vi "Calculate Curve Distance.vi"(9 "error in (no error)":errorcluster, 11 "Points":T1[](array[typedef])) -> (1 "error out":errorcluster, 2 "Length":dbl, 3 "Points Out":T1[](array[typedef]), 5 "Distance vs t":cluster{"t":dbl[], "Distance":dbl[]})   [LabVIEW 2019, in "Tool Path.lvclass"]
uses:
  Tool Path.lvclass
  Parse/PathCommands/Point.ctl
  Parse/PathCommands/PathCommands.lvclass
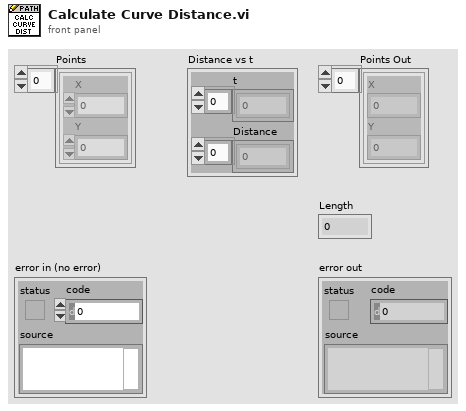
[diagram p1: front panel]
types:
  T1 = typedef "PathCommands.lvclass/Point.ctl" = cluster{"X":dbl, "Y":dbl}
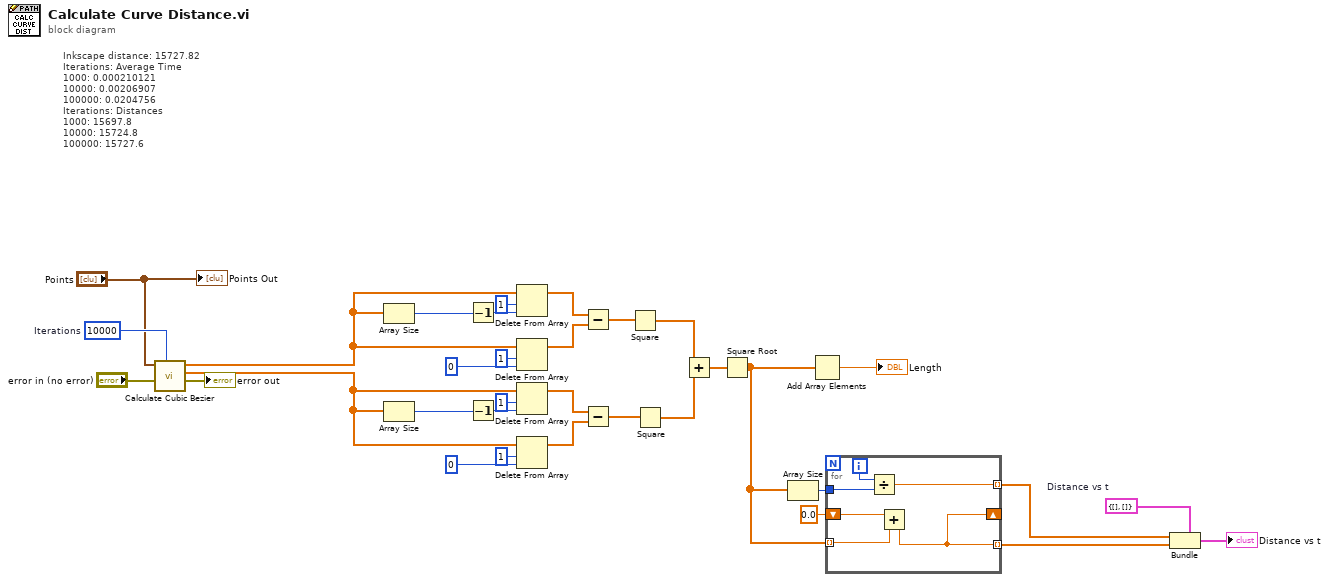
[diagram p0: block diagram]
diagram:
  w1 = cluster{"t":dbl[], "Distance":dbl[]} {"t"=[], "Distance"=[]}  # Distance vs t
  w19 = 10000  # Iterations
  # "Inkscape distance: 15727.82\nIterations: Average Time\n1000: 0.000210121\n10000: 0.00206907\n100000: 0.0204756\nIterations: Distances\n1000: 15697.8\n10000: 15724.8\n100000: 15727.6"
  n1 = call "Calculate Cubic Bezier.vi"("Iterations"=w19, "error in (no error)"="error in (no error)", "Points"="Points") -> ("error out"=→"error out":errorcluster, "Y"=w9:dbl[], "X"=w10:dbl[])  [unwired: 6 in]
  n2 = Array Size(array=w10) -> (size(s)=w33:i32)
  n3 = Array Size(array=w9) -> (size(s)=w23:i32)
  n4 = Decrement(x=w33) -> (x-1=w32:i32)
  n5 = Decrement(x=w23) -> (x-1=w24:i32)
  n6 = Delete From Array(array=w10, length=1, index=w32) -> (array with subset deleted=w18:dbl[])  [unwired: 1 out]
  n7 = Delete From Array(array=w10, length=1, index=0) -> (array with subset deleted=w17:dbl[])  [unwired: 1 out]
  n8 = Delete From Array(array=w9, length=1, index=w24) -> (array with subset deleted=w16:dbl[])  [unwired: 1 out]
  n9 = Delete From Array(array=w9, length=1, index=0) -> (array with subset deleted=w15:dbl[])  [unwired: 1 out]
  n10 = Subtract(x=w18, y=w17) -> (x-y=w28:dbl[])
  n11 = Subtract(x=w16, y=w15) -> (x-y=w22:dbl[])
  n12 = Square(x=w28) -> (x^2=w14:dbl[])
  n13 = Square(x=w22) -> (x^2=w13:dbl[])
  n14 = Add(x=w14, y=w13) -> (x+y=w21:dbl[])
  n15 = Square Root(x=w21) -> (sqrt(x)=w7:dbl[])
  n16 = Array Size(array=w7) -> (size(s)=w6:i32)
  n17 = Add Array Elements(numeric array=w7) -> (sum=→"Length":dbl)
  n18 = for {
    tunnel: w7 -> [w38] mode=indexing
    tunnel: w6 -> [w34]
    shift-right: [w36] -> _
    shift-left: 0.0 -> [w39]
    tunnel: [w36] -> w2 mode=indexing
    tunnel: [w37] -> w3 mode=indexing
    i -> [w35]
    n19 = Divide(x=w35, y=w34) -> (x/y=w37:dbl)
    n20 = Add(x=w39, y=w38) -> (x+y=w36:dbl)
  }
  n21 = Bundle(cluster=w1, "t"=w3, "Distance"=w2) -> (→"Distance vs t":cluster{"t":dbl[], "Distance":dbl[]})
  "Points Out" <- "Points"
